vi "Make VI Param(Read Batch Profile Advance Rsp).vi"(1 "pRsp":T1) -> (0 "Read Batch Profile Advance Rsp":T2)   [LabVIEW 8.6, in "Keyence LJ-V7000.lvlib"]
uses:
  Keyence LJ-V7000.lvlib
  Public/Clusters/Read Batch Profile Advance Rsp.ctl
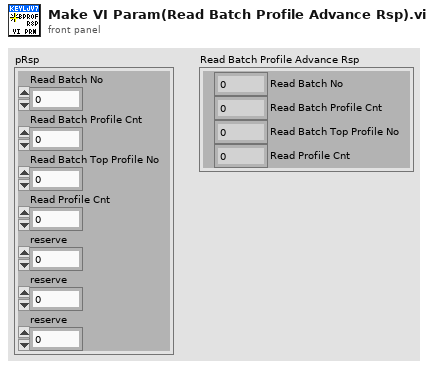
[diagram p1: front panel]
types:
  T1 = cluster{"Read Batch No":u32, "Read Batch Profile Cnt":u32, "Read Batch Top Profile No":u32, "Read Profile Cnt":u8, "reserve":u8, "reserve":u8, "reserve":u8}
  T2 = typedef "Keyence LJ-V7000.lvlib/Read Batch Profile Advance Rsp.ctl" = cluster{"Read Batch No":u32, "Read Batch Profile Cnt":u32, "Read Batch Top Profile No":u32, "Read Profile Cnt":u8}
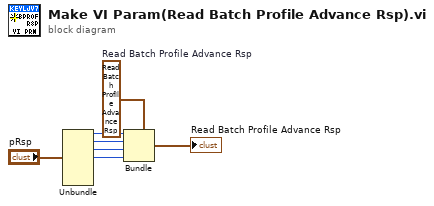
[diagram p0: block diagram]
diagram:
  w7 = T2 ?  # Read Batch Profile Advance Rsp
  n1 = Unbundle("pRsp") -> ("Read Batch No"=w5:u32, "Read Batch Profile Cnt"=w4:u32, "Read Batch Top Profile No"=w3:u32, "Read Profile Cnt"=w2:u8)  [unwired: 3 out]
  n2 = Bundle(cluster=w7, "Read Batch No"=w5, "Read Batch Profile Cnt"=w4, "Read Batch Top Profile No"=w3, "Read Profile Cnt"=w2) -> (→"Read Batch Profile Advance Rsp":T2)
